vi "QuinticHermiteSpline_New.vi"(8 "yFinalCtrlVector":dbl[](array[numeric]), 9 "yInitialCtrlVector":dbl[](array[numeric]), 10 "xFinalCtrlVector":dbl[](array[numeric]), 11 "XInitialCtrlVector":dbl[](array[numeric])) -> (0 "error out":errorcluster, 3 "QuinticHermiteSpline":T1)   [LabVIEW 2019, in "Trajectory_Library.lvlib"]
doc: "Constructs a quintic hermite spline with the specified control vectors. Each control vector contains into about the location of the point, its first derivative, and its second derivative.\n\nParameters: \n - xInitialControlVector The control vector for the initial point in the x dimension.\n - xFinalControlVector The control vector for the final point in the x dimension.\n - yInitialControlVector The control vector for the initial point in the y dimension.\n - yFinalControlVector The control vector for the final point in the y dimension.\n\nReturns:\n - QuinticHermiteSpline - The resulting spline\n - Error Out - The resulting error cluster"
uses:
  Trajectory_Library.lvlib
  SPLINE.ctl
  <vilib>/Analysis/Matrix/Datatypes/RealMatrix.ctl
  <vilib>/Analysis/Matrix/Numeric/Multiply/Multiply - RM,RM.vi
  <vilib>/Analysis/Matrix/NI_Matrix.lvlib
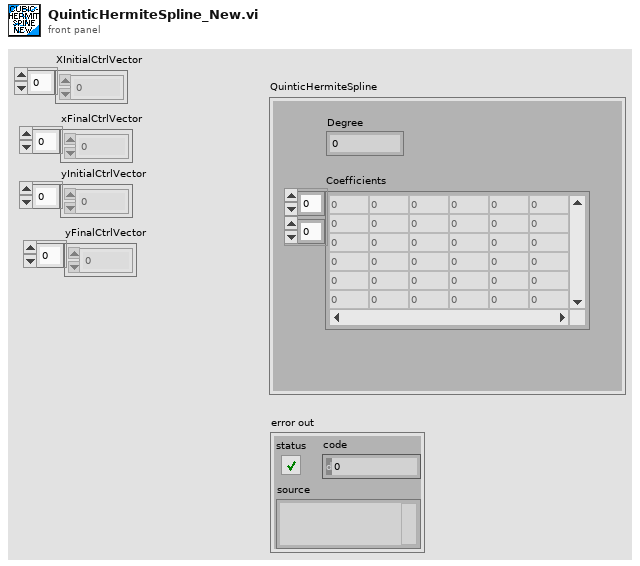
[diagram p1: front panel]
types:
  T1 = typedef "Trajectory_Library.lvlib/SPLINE.ctl" = cluster{"Degree":i32, "Coefficients":T2}
  T2 = typedef "NI_Matrix.lvlib/RealMatrix.ctl" = dbl[][]
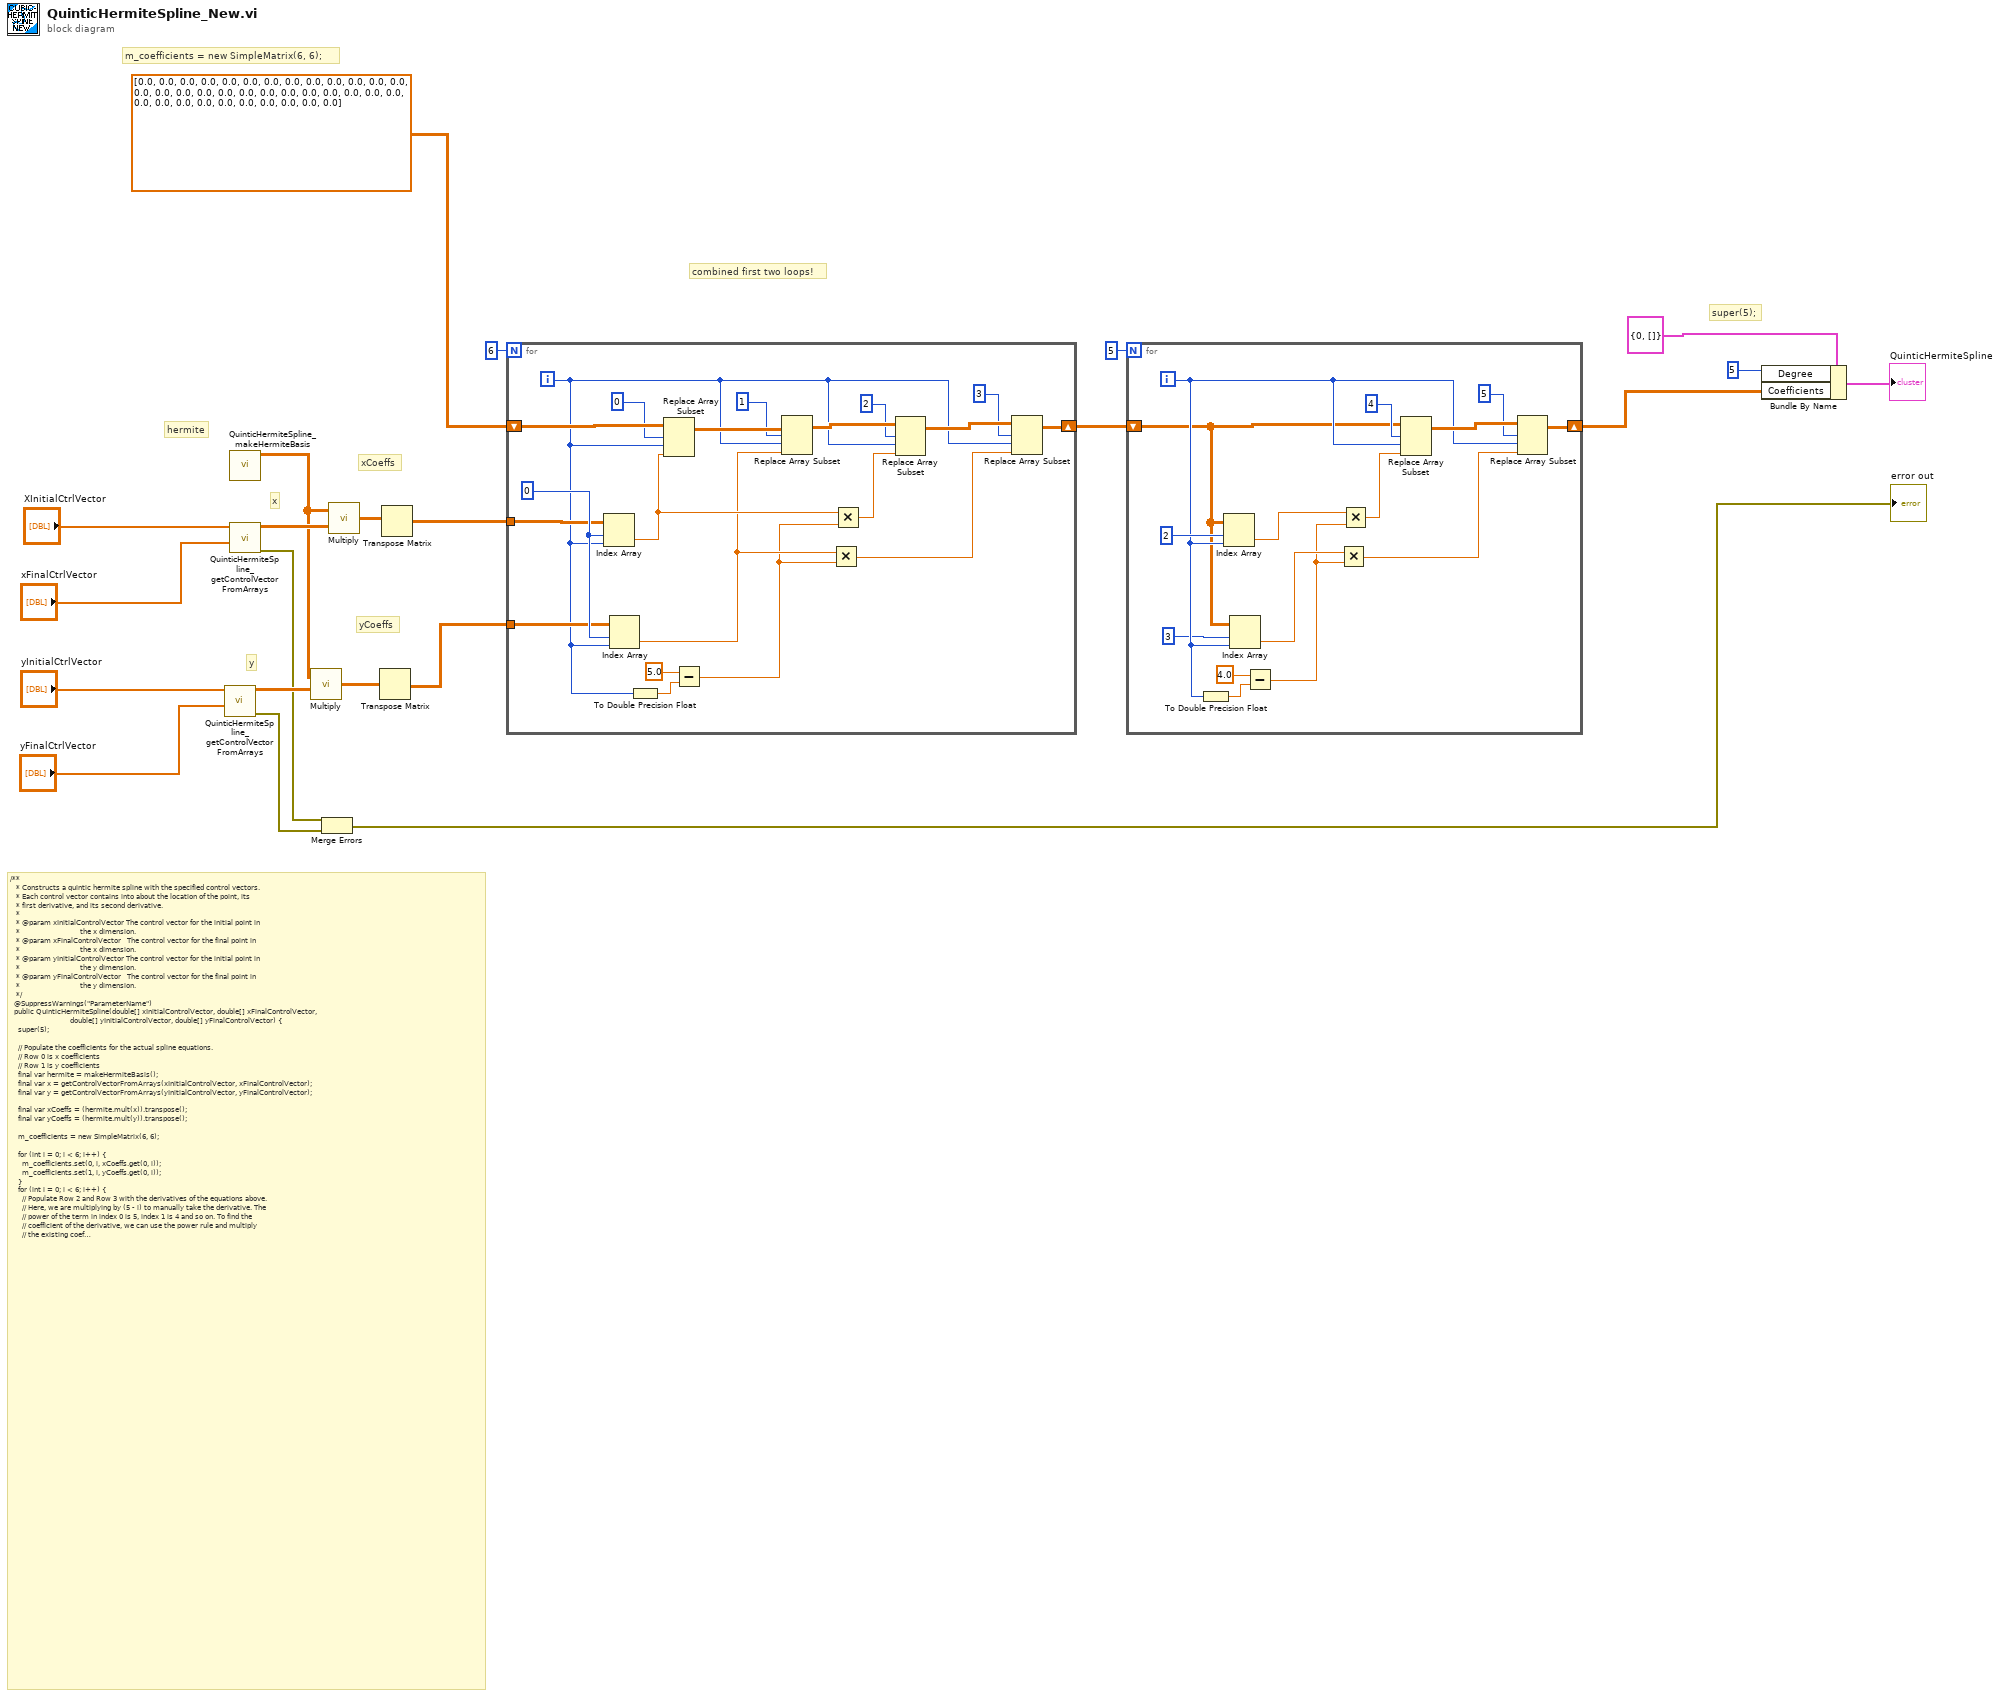
[diagram p0: block diagram]
diagram:
  # "combined first two loops!"
  # "yCoeffs"
  # "xCoeffs"
  # "m_coefficients = new SimpleMatrix(6, 6);"
  # "hermite"
  # "y"
  # "x"
  # "super(5);"
  # "/**\n   * Constructs a quintic hermite spline with the specified control vectors.\n   * Each control vector contains into about the location of the point, its\n   * first derivative, and its second derivative.\n   *\n   * @param xInitialControlVector The control vector for the initial point in\n   *                              the x dimension.\n   * @param xFinalControlVector   The control vector for the final point in\n   *                              the x dimension.\n   * @param yInitialControlVector The control vector for the initial point in\n   *                              the y dimension.\n   * @param yFinalControlVector   The control vector for the final point in\n   *                              the y dimension.\n   */\n  @SuppressWarnings(\"ParameterName\")\n  public QuinticHermiteSpline(double[] xInitialControlVector, double[] xFinalControlVector,\n                              double[] yInitialControlVector, double[] yFinalControlVector) {\n    super(5);\n\n    // Populate the coefficients for the actual spline equations.\n    // Row 0 is x coefficients\n    // Row 1 is y coefficients\n    final var hermite = makeHermiteBasis();\n    final var x = getControlVectorFromArrays(xInitialControlVector, xFinalControlVector);\n    final var y = getControlVectorFromArrays(yInitialControlVector, yFinalControlVector);\n\n    final var xCoeffs = (hermite.mult(x)).transpose();\n    final var yCoeffs = (hermite.mult(y)).transpose();\n\n    m_coefficients = new SimpleMatrix(6, 6);\n\n    for (int i = 0; i < 6; i++) {\n      m_coefficients.set(0, i, xCoeffs.get(0, i));\n      m_coefficients.set(1, i, yCoeffs.get(0, i));\n    }\n    for (int i = 0; i < 6; i++) {\n      // Populate Row 2 and Row 3 with the derivatives of the equations above.\n      // Here, we are multiplying by (5 - i) to manually take the derivative. The\n      // power of the term in index 0 is 5, index 1 is 4 and so on. To find the\n      // coefficient of the derivative, we can use the power rule and multiply\n      // the existing coefficient by its power.\n      m_coefficients.set(2, i, m_coefficients.get(0, i) * (5 - i));\n      m_coefficients.set(3, i, m_coefficients.get(1, i) * (5 - i));\n    }\n    for (int i = 0; i < 5; i++) {\n      // Then populate row 4 and 5 with the second derivatives.\n      // Here, we are multiplying by (4 - i) to manually take the derivative. The\n      // power of the term in index 0 is 4, index 1 is 3 and so on. To find the\n      // coefficient of the derivative, we can use the power rule and multiply\n      // the existing coefficient by its power.\n      m_coefficients.set(4, i, m_coefficients.get(2, i) * (4 - i));\n      m_coefficients.set(5, i, m_coefficients.get(3, i) * (4 - i));\n    }\n  }"
  n1 = call "QuinticHermiteSpline_getControlVectorFromArrays.vi"("finalVector"="yFinalCtrlVector", "initialVector"="yInitialCtrlVector") -> ("error out"=w4:errorcluster, "ControlVector"=w16:T2)  [unwired: 8 in]
  n2 = call "QuinticHermiteSpline_makeHermiteBasis.vi"() -> ("HermiteBasis"=w7:T2)  [unwired: 11 in]
  n3 = call "QuinticHermiteSpline_getControlVectorFromArrays.vi"("finalVector"="xFinalCtrlVector", "initialVector"="XInitialCtrlVector") -> ("error out"=w5:errorcluster, "ControlVector"=w17:T2)  [unwired: 8 in]
  n4 = call-poly <vilib>:"Multiply.vi"("Real Matrix B"=w16, "Real Matrix A"=w7) -> ("A * B"=w14:T2)
  n5 = Merge Errors(w5, w4) -> (→"error out":errorcluster)
  n6 = call-poly <vilib>:"Multiply.vi"("Real Matrix B"=w17, "Real Matrix A"=w7) -> ("A * B"=w15:T2)
  n7 = Transpose Matrix(1:w14) -> (0:w10:T2)
  n8 = Transpose Matrix(1:w15) -> (0:w11:T2)
  n9 = for {
    N: 6 -> [_]
    shift-right: [w39] -> w8
    shift-left: T2 [[0.0, 0.0, 0.0, 0.0, 0.0, 0.0], [0.0, 0.0, 0.0, 0.0, 0.0, 0.0], [0.0, 0.0, 0.0, 0.0, 0.0, 0.0], [0.0, 0.0, 0.0, 0.0, 0.0, 0.0], [0.0, 0.0, 0.0, 0.0, 0.0, 0.0], [0.0, 0.0, 0.0, 0.0, 0.0, 0.0]] ("HermiteBasis") -> [w42]
    tunnel: w11 -> [w34]
    tunnel: w10 -> [w33]
    i -> [w32]
    w35 = 0 ("index (row)")
    n10 = Index Array(array=w34, index (row)=w35, index (col)=w32) -> (element=w29:dbl)
    n11 = Index Array(array=w33, index (row)=w35, index (col)=w32) -> (element=w25:dbl)
    n12 = To Double Precision Float(number=w32) -> (double precision float=w31:dbl)
    n13 = Replace Array Subset(array=w42, new element=w29, index (row)=0 ("disabled index (row)"), index (col)=w32) -> (w41:T2)
    n14 = Subtract(x=5.0, y=w31) -> (x-y=w24:dbl)
    n15 = Replace Array Subset(array=w41, new element=w25, index (row)=1 ("disabled index (row)"), index (col)=w32) -> (w40:T2)
    n16 = Multiply(x=w25, y=w24) -> (x*y=w23:dbl)
    n17 = Multiply(x=w29, y=w24) -> (x*y=w26:dbl)
    n18 = Replace Array Subset(array=w40, new element=w26, index (row)=2 ("disabled index (row)"), index (col)=w32) -> (w38:T2)
    n19 = Replace Array Subset(array=w38, new element=w23, index (row)=3 ("disabled index (row)"), index (col)=w32) -> (w39:T2)
  }
  n20 = for {
    N: 5 -> [_]
    shift-right: [w57] -> w2
    shift-left: w8 -> [w43]
    i -> [w54]
    n21 = To Double Precision Float(number=w54) -> (double precision float=w53:dbl)
    n22 = Index Array(array=w43, index (row)=2, index (col)=w54) -> (element=w51:dbl)
    n23 = Index Array(array=w43, index (row)=3, index (col)=w54) -> (element=w47:dbl)
    n24 = Subtract(x=4.0, y=w53) -> (x-y=w46:dbl)
    n25 = Multiply ("Multiply.vi")(x=w47, y=w46) -> (x*y=w45:dbl)
    n26 = Multiply(x=w51, y=w46) -> (x*y=w48:dbl)
    n27 = Replace Array Subset(array=w43, new element=w48, index (row)=4 ("disabled index (row)"), index (col)=w54) -> (w56:T2)
    n28 = Replace Array Subset(array=w56, new element=w45, index (row)=5 ("disabled index (row)"), index (col)=w54) -> (w57:T2)
  }
  n29 = Bundle By Name(cluster=T1 {"Degree"=0, "Coefficients"=[]} ("SPLINE"), "Degree"=5 ("SPLINE.Degree"), "Coefficients"=w2) -> (→"QuinticHermiteSpline":T1)
